vi "hdt_build_stream_ort.vi"(11 "readyForOutput":bool[](array[boolean])=[FALSE, FALSE, FALSE, FALSE, FALSE, FALSE, FALSE]) -> (3 "dataStream":cluster{fxp<+/-,22,1>[], bool[]})   [LabVIEW 2016]
uses:
  <vilib>/rvi/Emulation/niFpgaEmulationIsFPGAContextNoSignature.vi
  <vilib>/rvi/Emulation/niFpgaSctlEmulationGetInTimedLoop.vi
  <vilib>/rvi/errors/niFpgaSetErrorForExecOnDevCompSimple.vi
  <vilib>/rvi/eio/common/nirviEmuReportErrorAndStop.vi
  <vilib>/rvi/DataTransferAndStorage/Container/Common/niFpgaContainerGetUniqueNameForEmu.vi
  <vilib>/rvi/FIFO/Fifo_Resource/nirvififoEmulationSetSize.vi
  <vilib>/rvi/FIFO/Fifo_Resource/nirviFifoEmulationQueueMgr.vi
  <instcachedir>/0/nirviFifoEmulationQueueMgr_E5CAEC123FF24DC58D834DCA3CDAA9B5.lvgen/nirviFifoEmulationQueueMgr_E5CAEC123FF24DC58D834DCA3CDAA9B5_003.vi
  <vilib>/Utility/error.llb/Clear Errors.vi
  <vilib>/rvi/FIFO/Fifo_Resource/nirvififoEmulationCreateLock.vi
  <vilib>/rvi/Emulation/niFpgaProcessEmulError.vi
  <vilib>/rvi/FIFO/Fifo_Resource/nirvififoEmulationObtainLock.vi
  <vilib>/rvi/FIFO/Fifo_Resource/nirvififoEmulationReleaseLock.vi
  <vilib>/rvi/occurrence/nirviWaitOnOccurrenceBase.vi
  <vilib>/rvi/errors/nirviReportUnexpectedCaseInternalError.vi
  <vilib>/rvi/errors/nirviReportUnexpectedCaseInternalError (U32).vi
  <instcachedir>/0/nirviFifoEmulationQueueMgr_E5CAEC123FF24DC58D834DCA3CDAA9B5.lvgen/nirviFifoEmulationQueueMgr_E5CAEC123FF24DC58D834DCA3CDAA9B5_001.vi
  <instcachedir>/0/nirviFifoEmulationQueueMgr_E5CAEC123FF24DC58D834DCA3CDAA9B5.lvgen/nirviFifoEmulationQueueMgr_E5CAEC123FF24DC58D834DCA3CDAA9B5_000.vi
  <instcachedir>/0/nirviFifoEmulationQueueMgr_E5CAEC123FF24DC58D834DCA3CDAA9B5.lvgen/nirviFifoEmulationQueueMgr_E5CAEC123FF24DC58D834DCA3CDAA9B5_014.vi
  <vilib>/rvi/DataTransferAndStorage/Container/XNode/niFpgaContainer.xnode
  <vilib>/rvi/FIFO/Fifo_Resource/nirvififoEmulationRead.vi
  <vilib>/rvi/FXPMathLib/FxpInterpret/XNode/nifxpmath_Interpret.xnode
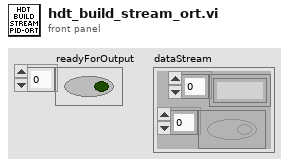
[diagram p1: front panel]
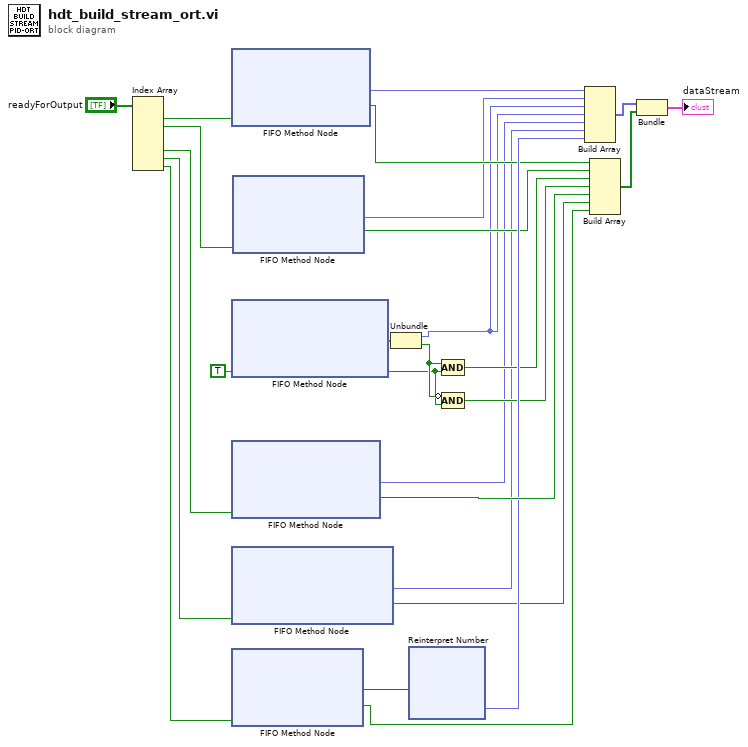
[diagram p0: block diagram]
diagram:
  n1 = Index Array(array="readyForOutput") -> (element #1=w23:bool, element #2=w24:bool, element #5=w27:bool, element #6=w26:bool, element #7=w25:bool)  [unwired: 7 in, 2 out]
  n2 = xnode ("FIFO Method Node")("Ready for Output"=w23) -> ("Element"=w18:fxp<+/-,22,1>, "Output Valid"=w10:bool)  [unwired: 1 in, 1 out]
  n3 = xnode ("FIFO Method Node")("Ready for Output"=TRUE) -> ("Element"=w4:cluster{"slope":fxp<+/-,22,1>, "forward":bool}, "Output Valid"=w2:bool)  [unwired: 1 in, 1 out]
  n4 = xnode ("FIFO Method Node")("Ready for Output"=w27) -> ("Element"=w8:fxp<+/-,22,1>, "Output Valid"=w21:bool)  [unwired: 1 in, 1 out]
  n5 = xnode ("FIFO Method Node")("Ready for Output"=w26) -> ("Element"=w9:fxp<+/-,18,1>, "Output Valid"=w14:bool)  [unwired: 1 in, 1 out]
  n6 = xnode ("FIFO Method Node")("Ready for Output"=w25) -> ("Element"=w5:i16, "Output Valid"=w22:bool)  [unwired: 1 in, 1 out]
  n7 = xnode ("FIFO Method Node")("Ready for Output"=w24) -> ("Element"=w6:fxp<+/-,22,1>, "Output Valid"=w11:bool)  [unwired: 1 in, 1 out]
  n8 = Unbundle(w4) -> ("slope"=w7:fxp<+/-,22,1>, "forward"=w3:bool)
  n9 = xnode "Reinterpret Number"("x"=w5) -> ("y"=w19:fxp<+/-,16,1>)
  n10 = Compound Arithmetic op=AND(w3, w2) -> (w12:bool)
  n11 = Compound Arithmetic op=AND(invert w3, w2) -> (w13:bool)
  n12 = Build Array(w18, w6, w7, w7, w8, w9, w19) -> (w15:fxp<+/-,22,1>[])
  n13 = Build Array(w10, w11, w12, w13, w21, w14, w22) -> (w16:bool[])
  n14 = Bundle(w15, w16) -> (→"dataStream":cluster{fxp<+/-,22,1>[], bool[]})  [unwired: 1 in]
